vi "Configure Tracking.vi"(8 "error in (no error)":errorcluster, 10 "Track Channel (0: 30V Channel)":T1 caption="Channel (0: +6V)" items=["30V/3A Channel", "30V/3A Channel", "5V/3A Channel"], 11 "VISA resource name":refnum<visa-resource-name>) -> (0 "error out":errorcluster, 3 "VISA resource name out":refnum<visa-resource-name>)   [LabVIEW 2020, in "RIGOL DP800 Series.lvlib"]
doc: "Configures the channel track function."
uses:
  <instrlib>/RIGOL DP800 Series/RIGOL DP800 Series.lvlib
  <instrlib>/RIGOL DP800 Series/Public/Channels.ctl
panel:
  in  "Enable?":bool
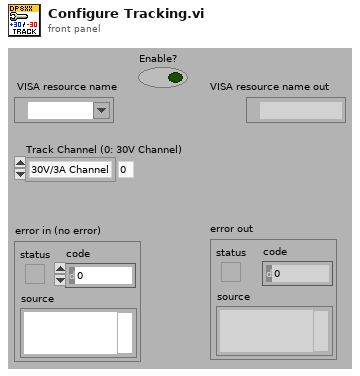
[diagram p1: front panel]
types:
  T1 = typedef "RIGOL DP800 Series.lvlib/Channels.ctl" = i32
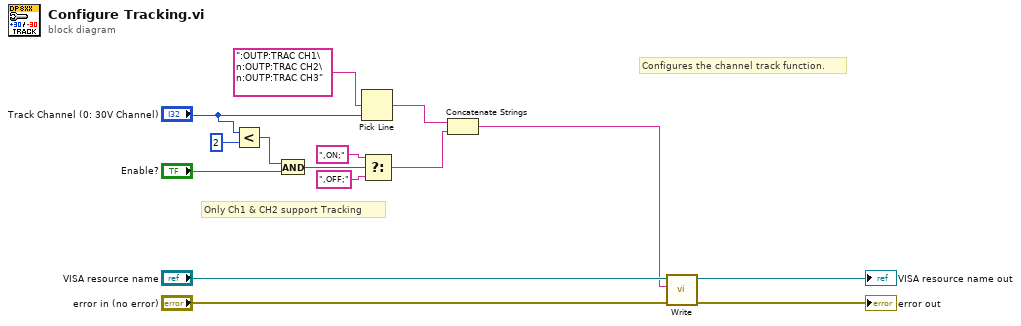
[diagram p0: block diagram]
diagram:
  # "Only Ch1 & CH2 support Tracking"
  # "Configures the channel track function."
  n1 = Less?(x="Track Channel (0: 30V Channel)", y=2) -> (x < y?=w4:bool)
  n2 = And(x=w4, y="Enable?") -> (x .and. y?=w2:bool)
  n3 = Pick Line(multi-line string=":OUTP:TRAC CH1\n:OUTP:TRAC CH2\n:OUTP:TRAC CH3", line index="Track Channel (0: 30V Channel)") -> (output string=w8:string)  [unwired: 1 out]
  n4 = Select(t=",ON;", s=w2, f=",OFF;") -> (s? t:f=w7:string)
  n5 = Concatenate Strings(w8, w7) -> (w6:string)
  n6 = call <instrlib>:"Write.vi"("error in (no error)"="error in (no error)", "Write Buffer (\"\")"=w6, "VISA resource name"="VISA resource name") -> ("error out"=→"error out":errorcluster, "VISA resource name out"=→"VISA resource name out":refnum<visa-resource-name>)  [unwired: 7 in]
